vi "Create I32Msg.vi"(8 "error in (no error)":errorcluster, 10 "Message Data":i32, 11 "Message Name":string) -> (0 "error out":errorcluster, 3 "I32Msg out":refnum<class "I32Msg.lvclass">)   [LabVIEW 2018, in "LapDog.Messaging.v3.NativeTypes.lvlib" / "I32Msg.lvclass"]
doc: "Returns an I32Msg object with the given name.\n\nThis method executes regardless of the error in state."
uses:
  I32Msg.lvclass
  T:/git/LapDog.Messaging/src/LapDog.Messaging/Message/Message.lvclass
  I32Msg.lvclass/I32Msg.ctl
  LapDog.Messaging/Message/Message.lvclass
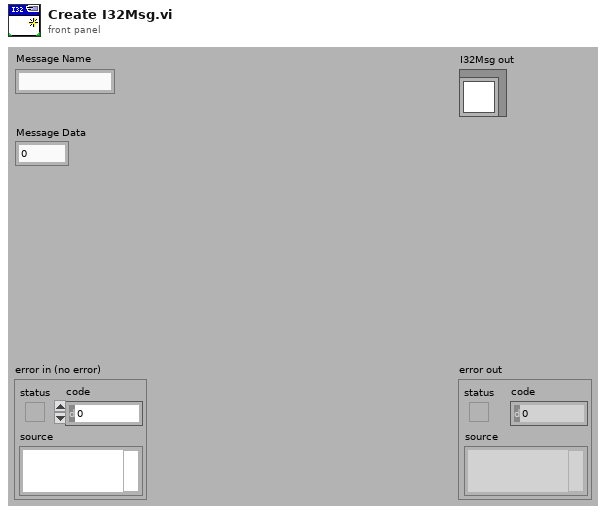
[diagram p1: front panel]
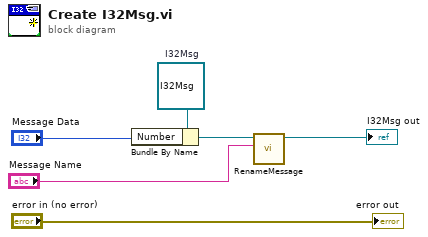
[diagram p0: block diagram]
diagram:
  w6 = refnum<class "I32Msg.lvclass"> refnum  # I32Msg
  n1 = Bundle By Name(cluster=w6, "Number"="Message Data") -> (w3:refnum<class "I32Msg.lvclass">)
  n2 = call "RenameMessage.vi"("Message Name"="Message Name", "Message in"=w3) -> ("Message out"=→"I32Msg out":refnum<class "I32Msg.lvclass">)  [unwired: 8 in, 1 out]
  "error out" <- "error in (no error)"
